vi "Actor Core.vi"(8 "error in":errorcluster, 11 "Car Wash Controller in":refnum<class "Car Wash Controller.lvclass">) -> (0 "error out":errorcluster, 3 "Actor out":refnum<class "Actor.lvclass">)   [LabVIEW 2019, in "Car Wash Controller.lvlib" / "Car Wash Controller.lvclass"]
doc: "(<B>Filename</B>: Actor Framework.lvlib:Actor.lvclass:Actor Core.vi)\n\nReceives messages to the actor, reacts to them, and initiates any error handling that may shut the actor down.\n\nDescendant classes may override this VI to append parallel tasks for the actor to complete while it handles messages. Overrides use the Call Parent Method node."
uses:
  Car Wash Controller.lvclass
  <vilib>/ActorFramework/Stop Msg/Stop Msg.lvclass
  <vilib>/ActorFramework/Actor/Actor.lvclass
  Car Wash Controller Messages/Set Lock Msg/Set Lock Msg.lvclass
  C:/Program Files (x86)/National Instruments/LabVIEW 2019/vi.lib/ActorFramework/Actor/Actor.lvclass
  Sim Configuration Database Actor/Sim Configuration Database Actor/Database Type.ctl
  Sim Configuration Database Actor/Sim Configuration Database Actor/Sim Configuration Database Actor.lvclass
  Sim Configuration Database Actor/Sim Configuration Database Actor/Record.ctl
  Vehicle Position Simulation Actor/Car Wash Controller/Station -Enum.ctl
  Vehicle Position Simulation Actor/Car Wash Controller/Vehicle Position Simulation Actor.lvclass
panel:
  in  "UI for DB":T4 {"Record"."Step Duration" format="%_5g"}
  # "SD7"
  # "SD6"
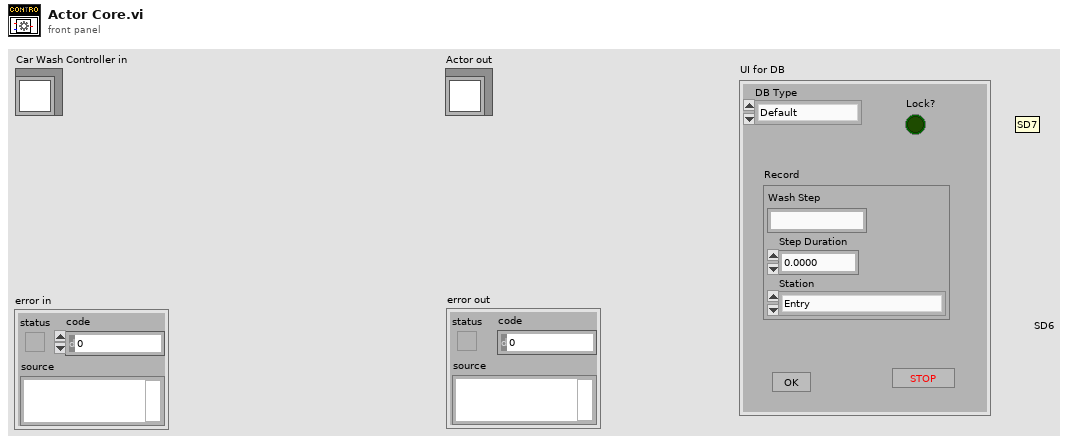
[diagram p1: front panel]
types:
  T1 = typedef "Sim Configuration Database Actor.lvlib/Sim Configuration Database Actor.lvclass/Database Type.ctl" = enum16{"Default", "Client"}
  T2 = typedef "Sim Configuration Database Actor.lvlib/Sim Configuration Database Actor.lvclass/Record.ctl" = cluster{"Wash Step":string, "Step Duration":dbl, "Station":T3}
  T3 = typedef "Vehicle Position Sinmulation Actor.lvlib/Vehicle Position Simulation Actor.lvclass/Station -Enum.ctl" = enum16{"Entry", "Station1", "Station2", "Station3", "Exit"}
  T4 = cluster{"DB Type":T1, "OK Button":bool, "stop":bool, "Record":T2, "Lock?":bool}
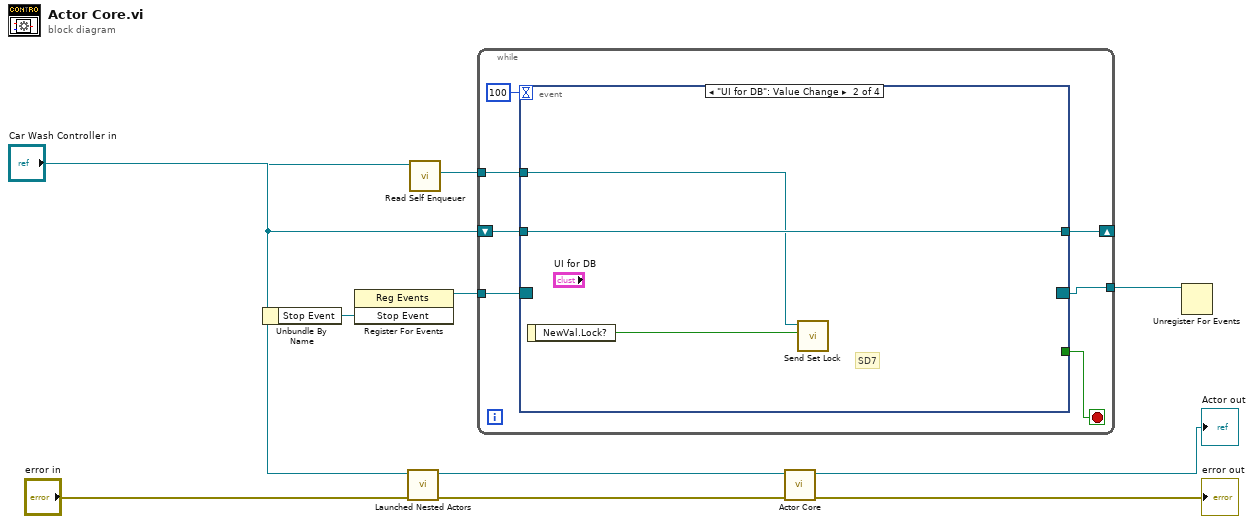
[diagram p0: block diagram]
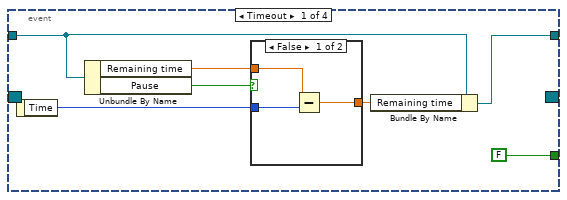
[diagram p2: hidden frame]
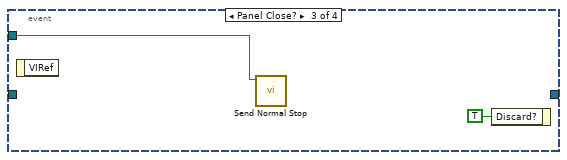
[diagram p4: hidden frame]
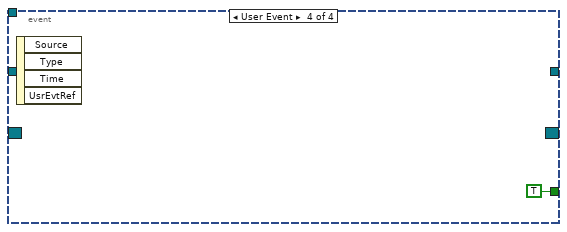
[diagram p5: hidden frame]
diagram:
  n1 = call "Launched Nested Actors.vi"("error in (no error)"="error in", "Car Wash Controller in"="Car Wash Controller in") -> ("error out"=w3:errorcluster, "Car Wash Controller out"=w1:refnum<class "Car Wash Controller.lvclass">)  [unwired: 8 in]
  n2 = Unbundle By Name(w1) -> ("Stop Event"=w4:refnum<user-event>)
  n3 = register-events(w4) -> (reference out=w7:refnum<event-registration>)  [unwired: 2 in, 1 out]
  n4 = call <vilib>:"Read Self Enqueuer.vi"("Actor"=w1) -> ("Self Enqueuer"=w5:refnum<class "Message Enqueuer.lvclass">)  [unwired: 10 in]
  n5 = while {
    tunnel: w7 -> [w16]
    tunnel: [w15] -> w6
    tunnel: w5 -> [w14]
    shift-right: [w11] -> _
    shift-left: w1 -> [w12]
    stop <- w17 stop-if-true
    n6 = event shown="[1] \"UI for DB\": Value Change" {
      selector: w16 -> [_ _ _ _]
      dyn-events: [_ _ _ _] -> w15
      timeout: 100 -> [_ _ _ _]
      tunnel: [FALSE _ _ TRUE] -> w17
      tunnel: w14 -> [_ w29 w32 _]
      tunnel: w12 -> [w21 w31 _ _]
      tunnel: [w23 w31 _ _] -> w11
      event Timeout {
        n7 = event-data() -> ("Time"=w22:u32)  [unwired: 1 in]
        n8 = Unbundle By Name(w21) -> ("Remaining time"=w20:dbl, "Pause"=w18:bool)
        n9 = case shown="False" w18 {
          tunnel: w22 -> [w27 _]
          tunnel: w20 -> [w26 w28]
          tunnel: [w25 w28] -> w19
          frame False {
            n10 = Subtract(x=w26, y=w27) -> (x-y=w25:dbl)
          }
          frame True {
          }
        }
        n11 = Bundle By Name(cluster=w21, "Remaining time"=w19) -> (w23:refnum<class "Car Wash Controller.lvclass">)
      }
      event "UI for DB": Value Change {
        # "SD7"
        n12 = event-data() -> ("NewVal.Lock?"=w30:bool)  [unwired: 1 in]
        n13 = call "Send Set Lock.vi"("Lock"=w30, "Message Enqueuer"=w29) -> ()  [unwired: 8 in, 2 out]
      }
      event Panel Close? {
        n14 = event-data() -> ()  [unwired: 1 in, 1 out]
        n15 = call <vilib>:"Send Normal Stop.vi"("Message Enqueuer"=w32) -> ()  [unwired: 10 in, 1 out]
        n16 = event-data("Discard?"=TRUE) -> ()  [unwired: 1 in, 1 out]
      }
      event User Event {
        n17 = event-data() -> ()  [unwired: 1 in, 4 out]
      }
    }
  }
  n18 = call-parent "Actor Core.vi"("error in"=w3, "Actor in"=w1) -> ("error out"=→"error out":errorcluster, "Actor out"=→"Actor out":refnum<class "Actor.lvclass">)  [unwired: 8 in]
  n19 = Unregister For Events(event registration refnum=w6) -> ()  [unwired: 1 in, 1 out]
